vi "Get Current Position.vi"(8 "error in (no error)":errorcluster, 10 "Axis":T1=enum."X", 11 "VISA in":refnum<visa-resource-name>) -> (0 "error out":errorcluster, 2 "position [internal units]":dbl, 3 "VISA out":refnum<visa-resource-name>)   [LabVIEW 2017, in "Drivers.lvlib" / "ASI TG-1000.lvlib"]
doc: "Queries the ASI controller for the current position of the specified axes; the equivalent of the WHERE command."
uses:
  ASI TG-1000.lvlib
  Utility/Axis Name.ctl
  Utility/Serial Response Syntax.ctl
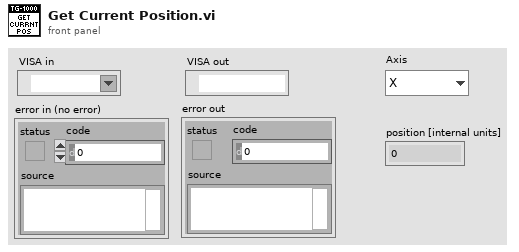
[diagram p1: front panel]
types:
  T1 = typedef "Drivers.lvlib/ASI TG-1000.lvlib/Axis Name.ctl" = enum8{"undefined", "A", "B", "C", "D", "E", "F", "G", "H", "I", "J", "K", "L", "M", "N", "O", "P", "Q", "R", "S", "T", "U", "V", "W", "X", "Y", "Z"}
  T2 = typedef "Drivers.lvlib/ASI TG-1000.lvlib/Serial Response Syntax.ctl" = enum16{":A then single line", "Single line, no :A", ":A or : then single line", ":A then single number", ":A or : then single number", ":A then <axis>= single number"}
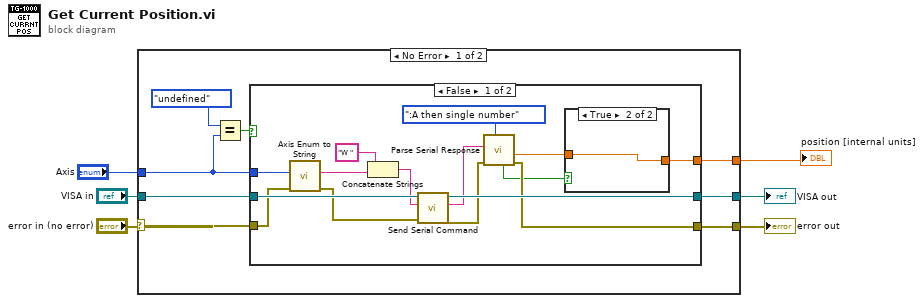
[diagram p0: block diagram]
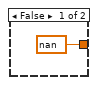
[diagram p2: hidden frame]
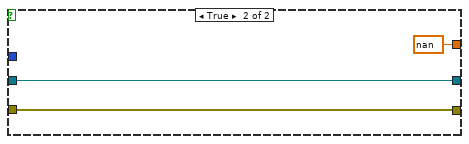
[diagram p3: hidden frame]
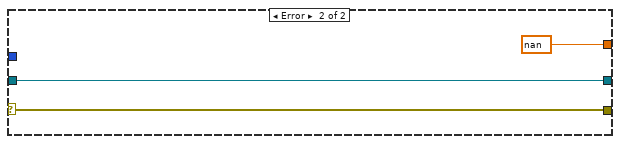
[diagram p4: hidden frame]
diagram:
  n1 = case shown="No Error" "error in (no error)" {
    selector: "error in (no error)" -> [w10 w37]
    tunnel: "VISA in" -> [w14 w36]
    tunnel: [w13 w36] -> w5
    tunnel: [w12 w37] -> w4
    tunnel: "Axis" -> [w8 _]
    tunnel: [w11 nan ("element")] -> w1
    frame No Error {
      n2 = Equal?(x=Axis_Name."undefined", y=w8) -> (x = y?=w9:bool)
      n3 = case shown="False" w9 {
        tunnel: w14 -> [w29 w33]
        tunnel: [w28 w33] -> w13
        tunnel: [w27 w34] -> w12
        tunnel: [w26 nan ("Parsed Numeric")] -> w11
        tunnel: w8 -> [w25 _]
        tunnel: w10 -> [w18 w34]
        frame False {
          n4 = call "Axis Enum to String.vi"("error in (no error)"=w18, "Axis Enum In"=w25) -> ("error out"=w17:errorcluster, "Axis String Out"=w20:string)  [unwired: 8 in]
          n5 = Concatenate Strings("W " ("Command"), w20) -> (w23:string)
          n6 = call "Send Serial Command.vi"("error in (no error)"=w17, "Command"=w23, "VISA in"=w29) -> ("error out"=w19:errorcluster, "Response"=w21:string, "VISA out"=w28:refnum<visa-resource-name>)  [unwired: 6 in]
          n7 = call "Parse Serial Response.vi"("Response Syntax"=Serial_Response_Syntax.":A then single number" ("Type of Response"), "error in (no error)"=w19, "Raw Response"=w21) -> ("error out"=w27:errorcluster, "Parsed Double"=w15:dbl, "As expected?"=w16:bool)  [unwired: 5 in, 1 out]
          n8 = case shown="True" w16 {
            tunnel: [nan ("default value 1") w31] -> w26
            tunnel: w15 -> [_ w31]
            frame False {
            }
            frame True {
            }
          }
        }
        frame True {
        }
      }
    }
    frame Error {
    }
  }
  "VISA out" <- w5
  "error out" <- w4
  "position [internal units]" <- w1
